vi "writeDBL.vi"(8 "error in (no error)":errorcluster, 10 "Input":dbl, 11 "M1M3SAL in":refnum<class "M1M3SAL.lvclass">) -> (0 "error out":errorcluster, 3 "M1M3SAL out":refnum<class "M1M3SAL.lvclass">)   [LabVIEW 2016, in "M1M3SupportCommunicator.lvlib" / "M1M3SAL.lvclass"]
uses:
  M1M3SAL.lvclass
  M1M3SAL.lvclass/M1M3SAL.ctl
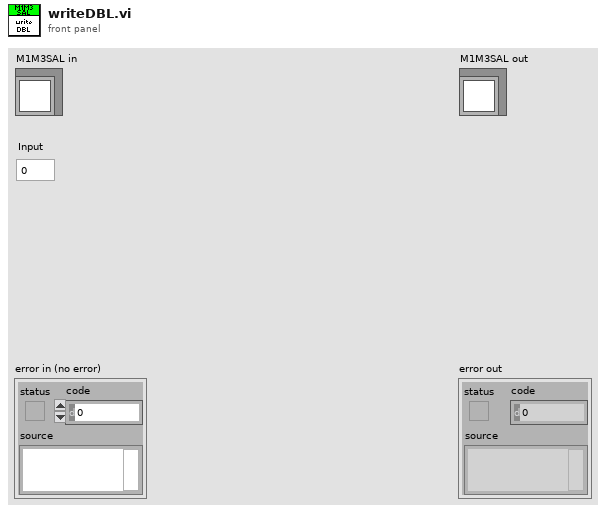
[diagram p1: front panel]
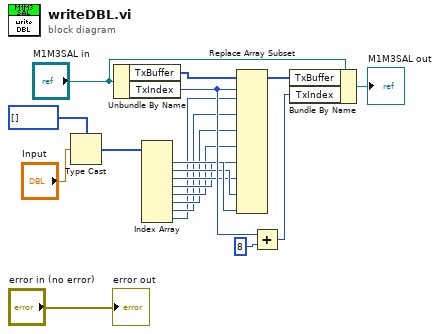
[diagram p0: block diagram]
diagram:
  n1 = Type Cast(type=u8[] [], x="Input") -> (*(type *) &x=w9:u8[])
  n2 = Unbundle By Name("M1M3SAL in") -> ("TxBuffer"=w17:u8[], "TxIndex"=w16:i32)
  n3 = Index Array(array=w9) -> (element #1=w8:u8, element #2=w7:u8, element #3=w6:u8, element #4=w5:u8, element #5=w4:u8, element #6=w3:u8, element #7=w2:u8, element #8=w1:u8)  [unwired: 8 in]
  n4 = Replace Array Subset(array=w17, new element #1=w1, index #1=w16, new element #2=w2, new element #3=w3, new element #4=w4, new element #5=w5, new element #6=w6, new element #7=w7, new element #8=w8) -> (w13:u8[])  [unwired: 7 in]
  n5 = Add(x=w16, y=8) -> (x+y=w14:i32)
  n6 = Bundle By Name(cluster="M1M3SAL in", "TxBuffer"=w13, "TxIndex"=w14) -> (→"M1M3SAL out":refnum<class "M1M3SAL.lvclass">)
  "error out" <- "error in (no error)"
